vi "SCCT Read XYZ Orientation.vi"(0 "Publisher In":refnum<class "Publisher.lvclass">, 1 "regular expression":string="Orientation Sensor</name><type>3</type><x>", 2 "search string/char (-)":string="</x>", 3 "regular expression 2":string="Orientation Sensor</name><type>3</type><x>", 5 "timeout in ms(0)":i32=100, 7 "search string/char (-) 3":string="</x>", 9 "regular expression 3":string="Orientation Sensor</name><type>3</type><x>", 11 "input cluster":errorcluster, 14 "search string/char (-) 2":string="</x>") -> (4 "Publisher Out":refnum<class "Publisher.lvclass">, 6 "x":string, 8 "y":string, 10 "XMLDocument":string, 12 "z":string, 13 "status":bool, 15 "error out 2":errorcluster)   [LabVIEW 2011]
uses:
  <vilib>/TOOLS FOR SMART MINDS/SCCT/Publisher/Publisher.lvclass
  <vilib>/TOOLS FOR SMART MINDS/SCCT/Publisher/Read XMLData.vi
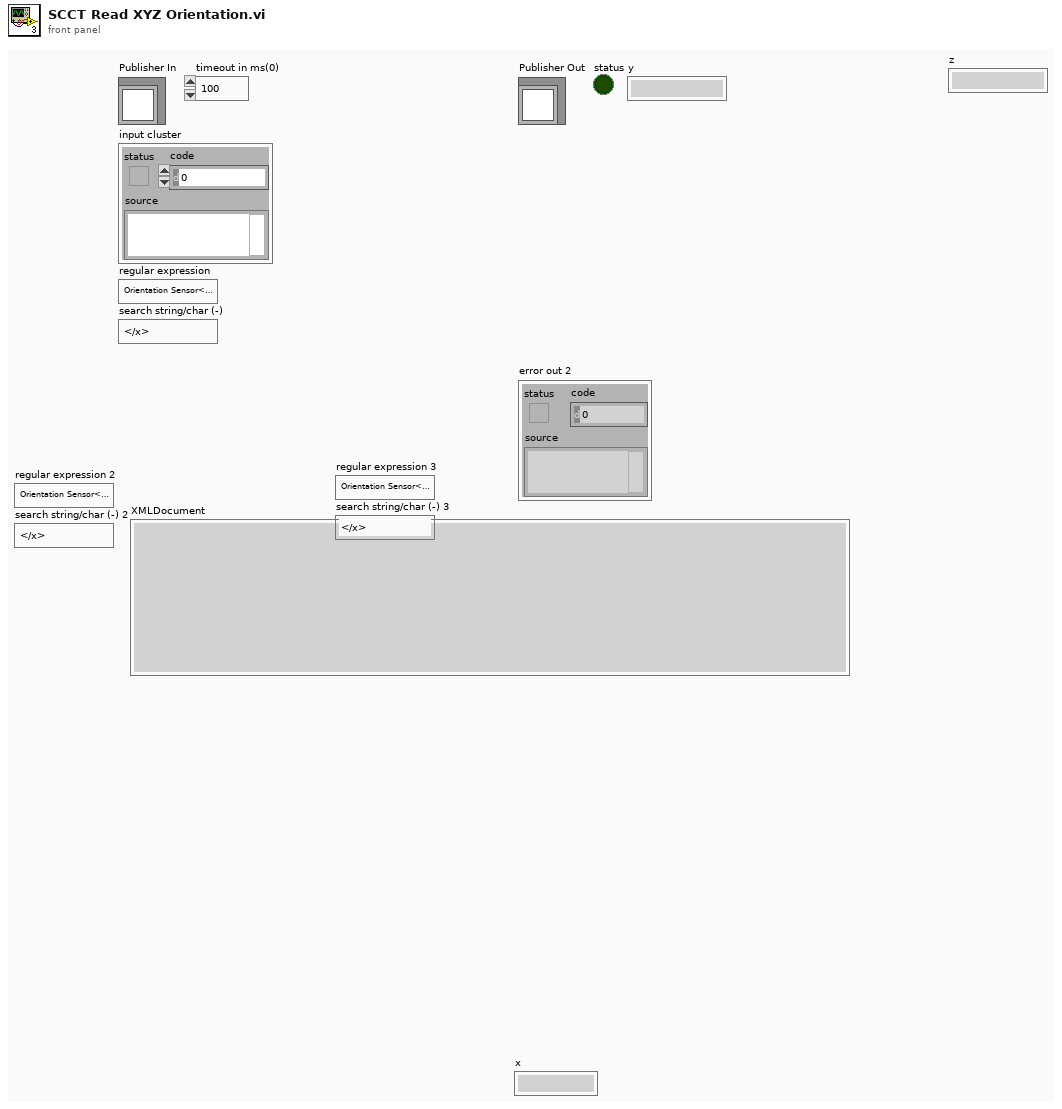
[diagram p1: front panel]
types:
  T1 = cluster{"timeStamp":timestamp, "value":cluster{"XMLDocument":string}, "senderAddress":string}
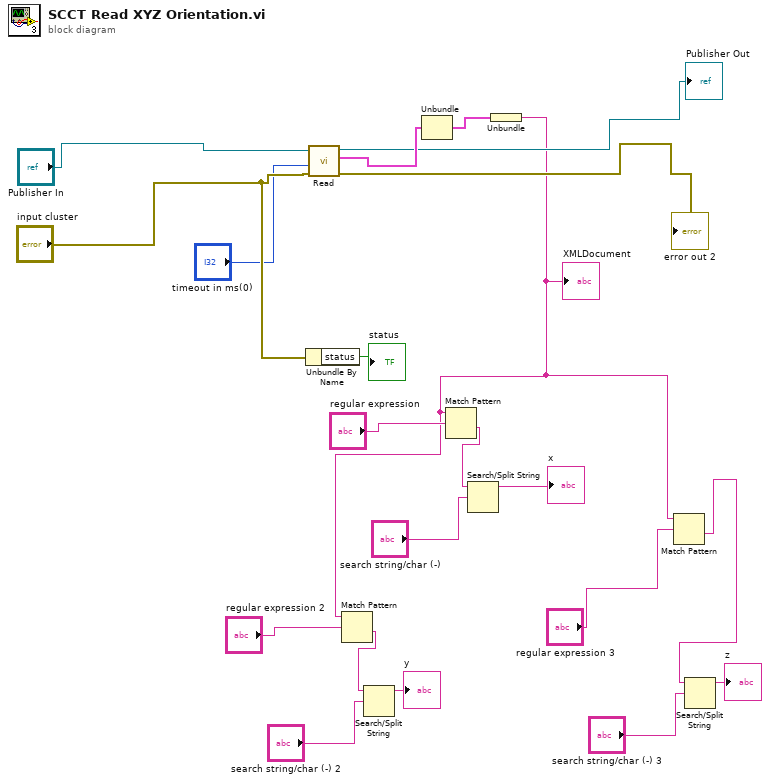
[diagram p0: block diagram]
diagram:
  n1 = Unbundle By Name("input cluster") -> ("status"=→"status":bool)
  n2 = call-poly <vilib>:"Read.vi"("error in (no error)"="input cluster", "timeout in ms(0)"="timeout in ms(0)", "Publisher In"="Publisher In") -> ("error out"=→"error out 2":errorcluster, "customXMLData"=w21:T1, "Publisher Out"=→"Publisher Out":refnum<class "Publisher.lvclass">)  [unwired: 4 in, 2 out]
  n3 = Unbundle(w21) -> ("value"=w20:cluster{"XMLDocument":string})  [unwired: 2 out]
  n4 = Unbundle(w20) -> ("XMLDocument"=w1:string)
  "XMLDocument" <- w1
  n5 = Match Pattern(string=w1, regular expression="regular expression 2") -> (after substring=w9:string)  [unwired: 1 in, 3 out]
  n6 = Search/Split String(string=w9, search string/char (-)="search string/char (-) 2") -> (substring before match=→"y":string)  [unwired: 1 in, 2 out]
  n7 = Match Pattern(string=w1, regular expression="regular expression") -> (after substring=w17:string)  [unwired: 1 in, 3 out]
  n8 = Search/Split String(string=w17, search string/char (-)="search string/char (-)") -> (substring before match=→"x":string)  [unwired: 1 in, 2 out]
  n9 = Match Pattern(string=w1, regular expression="regular expression 3") -> (after substring=w2:string)  [unwired: 1 in, 3 out]
  n10 = Search/Split String(string=w2, search string/char (-)="search string/char (-) 3") -> (substring before match=→"z":string)  [unwired: 1 in, 2 out]
